vi "GetBooksnAuthors.vi"(0 "reply string":string="150 Opening BINARY mode data connection for directory listing.\r\ntotal 89120\r\n-rw-r--r--  1 rbadmin  staff   11155 Jan 24 23:52 01242009235225_George Chan_Intro to LabVIEW.vi\r\n-rw-r--r--  1 rbadmin  staff  358797 Jan 24 23:52 01242009235225_George Chan_Intro to LabVIEW.zip\r\n-rw-r--r--  1 rbadmin  staff   11154 Jan 25 15:37 01252009153713_Dan Thayer_Intro to LabVIEW.vi\r\n-rw-r--r--  1 rbadmin  staff  368859 Jan 25 15:37 01252009153713_Dan Thayer_Intro to LabVIEW.zip\r\n-rw-r--r--  1 rbadmin  staff   11153 Jan 25 16:41 01252009164134_Dan Thayer_Intro to events.vi\r\n-rw-r--r--  1 rbadmin  staff  373332 Jan 25 16:41 01252009164134_Dan Thayer_Intro to events.zip\r\n-rw-r--r--  1 rbadmin  staff   11200 Jan 25 17:34 01252009173408_Robert Delean_Intro to events.vi\r\n-rw-r--r--  1 rbadmin  staff  337798 Jan 25 17:34 01252009173408_Robert Delean_Intro to events.zip\r\n-rw-r--r--  1 rbadmin  staff   11211 Jan 26 16:19 01262009161919_Alex Brindle_Intro to Events.vi\r\n-rw-r--r--  1 rbadmin  staff  353857 Jan 26 16:19 01262009161919_Alex Brindle_Intro to Events.zip\r\n-rw-r--r--  1 rbadmin  staff   11251 Jan 26 17:08 01262009170754_Alex Brindle_Introduction to LabVIEW.vi\r\n-rw-r--r--  1 rbadmin  staff  356261 Jan 26 17:07 01262009170754_Alex Brindle_Introduction to LabVIEW.zip\r\n-rw-r--r--  1 rbadmin  staff   11251 Jan 26 17:08 01262009170818_Alex Brindle_Introduction to LabVIEW.vi\r\n-rw-r--r--  1 rbadmin  staff  356261 Jan 26 17:08 01262009170818_Alex Brindle_Introduction to LabVIEW.zip\r\n-rw-r--r--  1 rbadmin  staff   11253 Jan 26 17:22 01262009172214_Alex Fernandes_Introduction to LabVIEW.vi\r\n-rw-r--r--  1 rbadmin  staff  355806 Jan 26 17:22 01262009172214_Alex Fernandes_Introduction to LabVIEW.zip\r\n-rw-r--r--  1 rbadmin  staff   11213 Jan 26 17:47 01262009174653_Alex Fernandes_Intro to Events.vi\r\n-rw-r--r--  1 rbadmin  staff  365514 Jan 26 17:46 01262009174653_Alex Fernandes_Intro to Events.zip\r\n-rw-r--r--  1 rbadmin  staff   11237 Jan 26 19:34 01262009193345_Ali Osman_Intro to LabVIEW.vi\r\n-rw-r--r--  1 rbadmin  staff  267924 Jan 26 19:33 01262009193345_Ali Osman_Intro to LabVIEW.zip\r\n-rw-r--r--  1 rbadmin  staff   11219 Jan 26 19:37 01262009193644_Michael Dawson-Haggerty_Intro to LabVIEW.vi\r\n-rw-r--r--  1 rbadmin  staff  268179 Jan 26 19:36 01262009193644_Michael Dawson-Haggerty_Intro to LabVIEW.zip\r\n-rw-r--r--  1 rbadmin  staff   11202 Jan 26 19:59 01262009195911_Michael Dawson-Haggerty_Intro to events.vi\r\n-rw-r--r--  1 rbadmin  staff  314967 Jan 26 19:59 01262009195911_Michael Dawson-Haggerty_Intro to events.zip\r\n-rw-r--r--  1 rbadmin  staff   11236 Jan 26 19:59 01262009195913_Ali Osman_Intro to events.vi\r\n-rw-r--r--  1 rbadmin  staff  315021 Jan 26 19:59 01262009195913_Ali Osman_Intro to events.zip\r\n-rw-r--r--  1 rbadmin  staff   11219 Jan 26 20:18 01262009201827_Timothy Roberts_Intro to LabVIEW.vi\r\n-rw-r--r--  1 rbadmin  staff  317960 Jan 26 20:18 01262009201827_Timothy Roberts_Intro to LabVIEW.zip\r\n-rw-r--r--  1 rbadmin  staff   11250 Jan 26 20:20 01262009202025_Timothy Roberts_Introduction to LabVIEW.vi\r\n-rw-r--r--  1 rbadmin  staff  317960 Jan 26 20:20 01262009202025_Timothy Roberts_Introduction to LabVIEW.zip\r\n-rw-r--r--  1 rbadmin  staff   11250 Jan 26 20:21 01262009202053_Timothy Roberts_Introduction to LabVIEW.vi\r\n-rw-r--r--  1 rbadmin  staff  317960 Jan 26 20:21 01262009202053_Timothy Roberts_Introduction to LabVIEW.zip\r\n-rw-r--r--  1 rbadmin  staff   11184 Jan 26 20:34 01262009203341_Nicole Slaughter_Intro to LabVIEW.vi\r\n-rw-r--r--  1 rbadmin  staff  353125 Jan 26 20:33 01262009203341_Nicole Slaughter_Intro to LabVIEW.zip\r\n-rw-r--r--  1 rbadmin  staff   11224 Jan 26 20:34 01262009203347_Arielle Fakhraee_Intro to LabVIEW.vi\r\n-rw-r--r--  1 rbadmin  staff  362150 Jan 26 20:34 01262009203347_Arielle Fakhraee_Intro to LabVIEW.zip\r\n-rw-r--r--  1 rbadmin  staff   11271 Jan 26 20:35 01262009203457_Arielle Fakhraee_Introduction to LabVIEW.vi\r\n-rw-r--r--  1 rbadmin  staff  362150 Jan 26 20:35 01262009203457_Arielle Fakhraee_Introduction to LabVIEW.zip\r\n-rw-r--r--  1 rbadmin  staff   11227 Jan 26 20:35 01262009203522_Nicole Slaughter_Introduction to LabVIEW.vi\r\n-rw-r--r--  1 rbadmin  staff  353125 Jan 26 20:35 01262009203522_Nicole Slaughter_Introduction to LabVIEW.zip\r\n-rw-r--r--  1 rbadmin  staff   11271 Jan 26 20:36 01262009203528_Arielle Fakhraee_Introduction to LabVIEW.vi\r\n-rw-r--r--  1 rbadmin  staff  362150 Jan 26 20:35 01262009203528_Arielle Fakhraee_Introduction to LabVIEW.zip\r\n-rw-r--r--  1 rbadmin  staff   11231 Jan 26 20:36 01262009203545_Nicole Slaughter_Introduction to LabVIEW.vi\r\n-rw-r--r--  1 rbadmin  staff  353125 Jan 26 20:35 01262009203545_Nicole Slaughter_Introduction to LabVIEW.zip\r\n-rw-r--r--  1 rbadmin  staff   11227 Jan 26 20:36 01262009203608_Nicole Slaughter_Introduction to LabVIEW.vi\r\n-rw-r--r--  1 rbadmin  staff  353125 Jan 26 20:36 01262009203608_Nicole Slaughter_Introduction to LabVIEW.zip\r\n-rw-r--r--  1 rbadmin  staff  321627 Jan 26 20:52 01262009205245_Lawrence Chan_Intro to LabVIEW.zip\r\n-rw-r--r--  1 rbadmin  staff  321661 Jan 26 20:53 01262009205323_Lawrence Chan_Introduction to LabVIEW.zip\r\n-rw-r--r--  1 rbadmin  staff   11248 Jan 26 20:53 01262009205326_Lawrence Chan_Introduction to LabVIEW.vi\r\n-rw-r--r--  1 rbadmin  staff  321661 Jan 26 20:53 01262009205326_Lawrence Chan_Introduction to LabVIEW.zip\r\n-rw-r--r--  1 rbadmin  staff   11201 Jan 26 20:53 01262009205339_Lawrence Chan_Intro to LabVIEW.vi\r\n-rw-r--r--  1 rbadmin  staff  321661 Jan 26 20:53 01262009205339_Lawrence Chan_Intro to LabVIEW.zip\r\n-rw-r--r--  1 rbadmin  staff   11279 Jan 26 21:06 01262009210629_Jeremiah Palmer_Intro to LabVIEW.vi\r\n-rw-r--r--  1 rbadmin  staff  269342 Jan 26 21:06 01262009210629_Jeremiah Palmer_Intro to LabVIEW.zip\r\n-rw-r--r--  1 rbadmin  staff  281166 Jan 26 21:15 01262009211511_William Murphy_Introduction to LabVIEW.zip\r\n-rw-r--r--  1 rbadmin  staff   11202 Jan 26 21:17 01262009211640_William Murphy_Intro to LabVIEW.vi\r\n-rw-r--r--  1 rbadmin  staff  281166 Jan 26 21:17 01262009211640_William Murphy_Intro to LabVIEW.zip\r\n-rw-r--r--  1 rbadmin  staff   11260 Jan 26 21:30 01262009213022_Drew Frankel_Intro to LabVIEW.vi\r\n-rw-r--r--  1 rbadmin  staff  269622 Jan 26 21:30 01262009213022_Drew Frankel_Intro to LabVIEW.zip\r\n-rw-r--r--  1 rbadmin  staff   11202 Jan 26 21:31 01262009213126_Derek Ricciuto_Intro to LabVIEW.vi\r\n-rw-r--r--  1 rbadmin  staff  258314 Jan 26 21:31 01262009213126_Derek Ricciuto_Intro to LabVIEW.zip\r\n-rw-r--r--  1 rbadmin  staff   11155 Jan 26 21:33 01262009213250_Ben Fichera_Intro to LabVIEW.vi\r\n-rw-r--r--  1 rbadmin  staff  264719 Jan 26 21:33 01262009213250_Ben Fichera_Intro to LabVIEW.zip\r\n-rw-r--r--  1 rbadmin  staff   11254 Jan 26 21:45 01262009214517_Timothy Roberts_Introduction to LabVIEW.vi\r\n-rw-r--r--  1 rbadmin  staff  317960 Jan 26 21:45 01262009214517_Timothy Roberts_Introduction to LabVIEW.zip\r\n-rw-r--r--  1 rbadmin  staff   11210 Jan 26 21:46 01262009214556_Timothy Roberts_Intro to Events.vi\r\n-rw-r--r--  1 rbadmin  staff  361042 Jan 26 21:46 01262009214556_Timothy Roberts_Intro to Events.zip\r\n-rw-r--r--  1 rbadmin  staff   11206 Jan 26 21:48 01262009214743_Timothy Roberts_Intro to events.vi\r\n-rw-r--r--  1 rbadmin  staff  361042 Jan 26 21:47 01262009214743_Timothy Roberts_Intro to events.zip\r\n-rw-r--r--  1 rbadmin  staff   11263 Jan 26 22:13 01262009221347_Drew Frankel_Intro to events.vi\r\n-rw-r--r--  1 rbadmin  staff  312829 Jan 26 22:13 01262009221347_Drew Frankel_Intro to events.zip\r\n-rw-r--r--  1 rbadmin  staff   11205 Jan 26 22:14 01262009221419_Derek Ricciuto_Intro to events.vi\r\n-rw-r--r--  1 rbadmin  staff  312573 Jan 26 22:14 01262009221419_Derek Ricciuto_Intro to events.zip\r\n-rw-r--r--  1 rbadmin  staff   11138 Jan 26 22:27 01262009222615_Ben Fichera_Intro to events.vi\r\n-rw-r--r--  1 rbadmin  staff  314194 Jan 26 22:26 01262009222615_Ben Fichera_Intro to events.zip\r\n-rw-r--r--  1 rbadmin  staff   11205 Jan 26 22:44 01262009224413_William Murphy_Intro to events.vi\r\n-rw-r--r--  1 rbadmin  staff  351616 Jan 26 22:44 01262009224413_William Murphy_Intro to events.zip\r\n-rw-r--r--  1 rbadmin  staff   11202 Jan 26 23:01 01262009230112_Courtney Mario_Intro to LabVIEW.vi\r\n-rw-r--r--  1 rbadmin  staff  353710 Jan 26 23:01 01262009230112_Courtney Mario_Intro to LabVIEW.zip\r\n-rw-r--r--  1 rbadmin  staff   11303 Jan 26 23:40 01262009234020_Austin Hsiao_Introduction to LabVIEW.vi\r\n-rw-r--r--  1 rbadmin  staff  283436 Jan 26 23:40 01262009234020_Austin Hsiao_Introduction to LabVIEW.zip\r\n-rw-r--r--  1 rbadmin  staff   11303 Jan 26 23:41 01262009234046_Austin Hsiao_Introduction to LabVIEW.vi\r\n-rw-r--r--  1 rbadmin  staff  283436 Jan 26 23:40 01262009234046_Austin Hsiao_Introduction to LabVIEW.zip\r\n-rw-r--r--  1 rbadmin  staff   11263 Jan 26 23:59 01262009235852_Austin Hsiao_Intro to Events.vi\r\n-rw-r--r--  1 rbadmin  staff  321775 Jan 26 23:59 01262009235852_Austin Hsiao_Intro to Events.zip\r\n-rw-r--r--  1 rbadmin  staff   11266 Jan 27 00:18 01272009001756_Jeremiah Palmer_Intro to events.vi\r\n-rw-r--r--  1 rbadmin  staff  320589 Jan 27 00:18 01272009001756_Jeremiah Palmer_Intro to events.zip\r\n-rw-r--r--  1 rbadmin  staff   11185 Jan 27 01:26 01272009012614_Timothy Li_Intro to Events.vi\r\n-rw-r--r--  1 rbadmin  staff  318752 Jan 27 01:26 01272009012614_Timothy Li_Intro to Events.zip\r\n-rw-r--r--  1 rbadmin  staff   11189 Jan 27 01:42 01272009014223_Taeil Kwak_Intro to events.vi\r\n-rw-r--r--  1 rbadmin  staff  345487 Jan 27 01:42 01272009014223_Taeil Kwak_Intro to events.zip\r\n-rw-r--r--  1 rbadmin  staff   11229 Jan 27 01:52 01272009015247_Timothy Li_Introduction to LabVIEW.vi\r\n-rw-r--r--  1 rbadmin  staff  305926 Jan 27 01:52 01272009015247_Timothy Li_Introduction to LabVIEW.zip\r\n-rw-r--r--  1 rbadmin  staff   11229 Jan 27 01:52 01272009015250_Timothy Li_Introduction to LabVIEW.vi\r\n-rw-r--r--  1 rbadmin  staff  305926 Jan 27 01:52 01272009015250_Timothy Li_Introduction to LabVIEW.zip\r\n-rw-r--r--  1 rbadmin  staff  269378 Jan 27 02:00 01272009020000_Taeil Kwak_Intro to LabVIEW.zip\r\n-rw-r--r--  1 rbadmin  staff   11202 Jan 27 02:10 01272009021016_Courtney Mario_Intro to LabVIEW.vi\r\n-rw-r--r--  1 rbadmin  staff  361928 Jan 27 02:10 01272009021016_Courtney Mario_Intro to LabVIEW.zip\r\n-rw-r--r--  1 rbadmin  staff   11260 Jan 27 04:26 01272009042554_Hannes Daepp_Intro to LabVIEW.vi\r\n-rw-r--r--  1 rbadmin  staff  291101 Jan 27 04:26 01272009042554_Hannes Daepp_Intro to LabVIEW.zip\r\n-rw-r--r--  1 rbadmin  staff   11263 Jan 27 04:32 01272009043213_Hannes Daepp_Intro to events.vi\r\n-rw-r--r--  1 rbadmin  staff  320888 Jan 27 04:32 01272009043213_Hannes Daepp_Intro to events.zip\r\n-rw-r--r--  1 rbadmin  staff   11157 Jan 27 10:09 01272009070920_Andres Cabrera_Intro to Events.vi\r\n-rw-r--r--  1 rbadmin  staff  363534 Jan 27 10:09 01272009070920_Andres Cabrera_Intro to Events.zip\r\n-rw-r--r--  1 rbadmin  staff   11161 Jan 27 10:10 01272009070956_Andres Cabrera_Intro to Events.vi\r\n-rw-r--r--  1 rbadmin  staff  363534 Jan 27 10:10 01272009070956_Andres Cabrera_Intro to Events.zip\r\n-rw-r--r--  1 rbadmin  staff   11157 Jan 27 08:48 01272009084805_Chris Rogers_Problem 1.vi\r\n-rw-r--r--  1 rbadmin  staff  304750 Jan 27 08:48 01272009084805_Chris Rogers_Problem 1.zip\r\n-rw-r--r--  1 rbadmin  staff   11286 Jan 27 09:46 01272009094540_Christopher Martin_Intro to LabVIEW.vi\r\n-rw-r--r--  1 rbadmin  staff  283893 Jan 27 09:45 01272009094540_Christopher Martin_Intro to LabVIEW.zip\r\n-rw-r--r--  1 rbadmin  staff   11285 Jan 27 09:46 01272009094616_Christopher Martin_Intro to events.vi\r\n-rw-r--r--  1 rbadmin  staff  318735 Jan 27 09:46 01272009094616_Christopher Martin_Intro to events.zip\r\n-rw-r--r--  1 rbadmin  staff   11205 Jan 27 12:49 01272009094837_Andres Cabrera_Introduction to LabVIEW.vi\r\n-rw-r--r--  1 rbadmin  staff  288050 Jan 27 12:48 01272009094837_Andres Cabrera_Introduction to LabVIEW.zip\r\n-rw-r--r--  1 rbadmin  staff   11205 Jan 27 12:49 01272009094916_Andres Cabrera_Introduction to LabVIEW.vi\r\n-rw-r--r--  1 rbadmin  staff  288050 Jan 27 12:49 01272009094916_Andres Cabrera_Introduction to LabVIEW.zip\r\n-rw-r--r--  1 rbadmin  staff   11247 Jan 27 13:29 01272009132901_Steve McHugh_Introduction to LabVIEW.vi\r\n-rw-r--r--  1 rbadmin  staff  304519 Jan 27 13:29 01272009132901_Steve McHugh_Introduction to LabVIEW.zip\r\n-rw-r--r--  1 rbadmin  staff   11247 Jan 27 13:29 01272009132924_Steve McHugh_Introduction to LabVIEW.vi\r\n-rw-r--r--  1 rbadmin  staff  304519 Jan 27 13:29 01272009132924_Steve McHugh_Introduction to LabVIEW.zip\r\n-rw-r--r--  1 rbadmin  staff   11247 Jan 27 13:30 01272009132947_Steve McHugh_Introduction to LabVIEW.vi\r\n-rw-r--r--  1 rbadmin  staff  304519 Jan 27 13:29 01272009132947_Steve McHugh_Introduction to LabVIEW.zip\r\n-rw-r--r--  1 rbadmin  staff   11181 Jan 27 14:34 01272009143348_Rachel Yu_Intro to LabVIEW.vi\r\n-rw-r--r--  1 rbadmin  staff  352379 Jan 27 14:34 01272009143348_Rachel Yu_Intro to LabVIEW.zip\r\n-rw-r--r--  1 rbadmin  staff   11180 Jan 27 14:35 01272009143512_Rachel Yu_Intro to events.vi\r\n-rw-r--r--  1 rbadmin  staff  360969 Jan 27 14:35 01272009143512_Rachel Yu_Intro to events.zip\r\n-rw-r--r--  1 rbadmin  staff   11203 Jan 27 14:39 01272009143930_Steve McHugh_Intro to events.vi\r\n-rw-r--r--  1 rbadmin  staff  378401 Jan 27 14:39 01272009143930_Steve McHugh_Intro to events.zip\r\n-rw-r--r--  1 rbadmin  staff   11201 Jan 27 15:49 01272009154908_Robert Delean_Intro to LabVIEW.vi\r\n-rw-r--r--  1 rbadmin  staff  321661 Jan 27 15:49 01272009154908_Robert Delean_Intro to LabVIEW.zip\r\n-rw-r--r--  1 rbadmin  staff   11204 Jan 27 16:15 01272009161523_Lawrence Chan_Intro to events.vi\r\n-rw-r--r--  1 rbadmin  staff  339180 Jan 27 16:15 01272009161523_Lawrence Chan_Intro to events.zip\r\n-rw-r--r--  1 rbadmin  staff   11187 Jan 27 16:32 01272009163211_Nicole Slaughter_Intro to Events.vi\r\n-rw-r--r--  1 rbadmin  staff  397876 Jan 27 16:32 01272009163211_Nicole Slaughter_Intro to Events.zip\r\n-rw-r--r--  1 rbadmin  staff   11183 Jan 27 16:33 01272009163240_Nicole Slaughter_Intro to events.vi\r\n-rw-r--r--  1 rbadmin  staff  397876 Jan 27 16:32 01272009163240_Nicole Slaughter_Intro to events.zip\r\n-rw-r--r--  1 rbadmin  staff   11201 Jan 27 17:41 01272009174122_Allyssa Alair_Intro to LabVIEW.vi\r\n-rw-r--r--  1 rbadmin  staff  268165 Jan 27 17:41 01272009174122_Allyssa Alair_Intro to LabVIEW.zip\r\n-rw-r--r--  1 rbadmin  staff   11223 Jan 27 18:31 01272009183051_Arielle Fakhraee_Intro to events.vi\r\n-rw-r--r--  1 rbadmin  staff  344835 Jan 27 18:31 01272009183051_Arielle Fakhraee_Intro to events.zip\r\n-rw-r--r--  1 rbadmin  staff   11204 Jan 27 19:06 01272009190603_Allyssa Alair_Intro to events.vi\r\n-rw-r--r--  1 rbadmin  staff  341333 Jan 27 19:06 01272009190603_Allyssa Alair_Intro to events.zip\r\n-rw-r--r--  1 rbadmin  staff   11256 Jan 27 19:41 01272009194048_Lindsay Wray_Intro to LabVIEW.vi\r\n-rw-r--r--  1 rbadmin  staff  299707 Jan 27 19:41 01272009194048_Lindsay Wray_Intro to LabVIEW.zip\r\n-rw-r--r--  1 rbadmin  staff   11260 Jan 27 19:44 01272009194344_Lindsay Wray_Intro to events1.vi\r\n-rw-r--r--  1 rbadmin  staff  320787 Jan 27 19:43 01272009194344_Lindsay Wray_Intro to events1.zip\r\n-rw-r--r--  1 rbadmin  staff   11160 Jan 27 20:52 01272009205145_Martin Rosas_Intro to LabVIEW.vi\r\n-rw-r--r--  1 rbadmin  staff  282345 Jan 27 20:51 01272009205145_Martin Rosas_Intro to LabVIEW.zip\r\n-rw-r--r--  1 rbadmin  staff   11184 Jan 27 21:13 01272009211333_Michael Stefaniak_Intro to events.vi\r\n-rw-r--r--  1 rbadmin  staff  317892 Jan 27 21:13 01272009211333_Michael Stefaniak_Intro to events.zip\r\n-rw-r--r--  1 rbadmin  staff  302248 Jan 28 13:20 01282009131958_Winston Lee_Intro to Events.zip\r\n-rw-r--r--  1 rbadmin  staff   11230 Jan 28 13:20 01282009132011_Winston Lee_Introduction to LabVIEW.vi\r\n-rw-r--r--  1 rbadmin  staff  263259 Jan 28 13:20 01282009132011_Winston Lee_Introduction to LabVIEW.zip\r\n-rw-r--r--  1 rbadmin  staff   11254 Jan 29 01:01 01292009010116_Jeremy Fryer-Biggs_Intro to LabVIEW.vi\r\n-rw-r--r--  1 rbadmin  staff  307078 Jan 29 01:01 01292009010116_Jeremy Fryer-Biggs_Intro to LabVIEW.zip\r\n-rw-r--r--  1 rbadmin  staff   11253 Jan 29 01:02 01292009010157_Jeremy Fryer-Biggs_Intro to events.vi\r\n-rw-r--r--  1 rbadmin  staff  373999 Jan 29 01:02 01292009010157_Jeremy Fryer-Biggs_Intro to events.zip\r\n-rw-r--r--  1 rbadmin  staff   11127 Jan 29 11:42 01292009084157_Andres Cabrera_Problem 1.vi\r\n-rw-r--r--  1 rbadmin  staff  319495 Jan 29 11:42 01292009084157_Andres Cabrera_Problem 1.zip\r\n-rw-r--r--  1 rbadmin  staff   11171 Jan 29 11:23 01292009112342_Derek Ricciuto_Problem 1.vi\r\n-rw-r--r--  1 rbadmin  staff  329882 Jan 29 11:23 01292009112342_Derek Ricciuto_Problem 1.zip\r\n-rw-r--r--  1 rbadmin  staff   11171 Jan 29 11:24 01292009112354_Courtney Mario_Problem 1.vi\r\n-rw-r--r--  1 rbadmin  staff  329829 Jan 29 11:24 01292009112354_Courtney Mario_Problem 1.zip\r\n-rw-r--r--  1 rbadmin  staff   11138 Jan 29 11:26 01292009112555_Michael Stefaniak_Problem 1.vi\r\n-rw-r--r--  1 rbadmin  staff  313818 Jan 29 11:26 01292009112555_Michael Stefaniak_Problem 1.zip\r\n-rw-r--r--  1 rbadmin  staff   11234 Jan 29 11:32 01292009113249_Thomas Williamson_Problem 1.vi\r\n-rw-r--r--  1 rbadmin  staff  310150 Jan 29 11:32 01292009113249_Thomas Williamson_Problem 1.zip\r\n-rw-r--r--  1 rbadmin  staff  317133 Jan 29 11:39 01292009113932_Lenny Paritsky_Problem 1.zip\r\n-rw-r--r--  1 rbadmin  staff  317133 Jan 29 11:39 01292009113944_Lenny Paritsky_Problem 1.zip\r\n-rw-r--r--  1 rbadmin  staff  317133 Jan 29 11:40 01292009113956_Lenny Paritsky_Problem 1.zip\r\n-rw-r--r--  1 rbadmin  staff  317133 Jan 29 11:40 01292009114017_Lenny Paritsky_Problem 1.zip\r\n-rw-r--r--  1 rbadmin  staff   11176 Jan 29 11:40 01292009114032_Timothy Roberts_Problem 1.vi\r\n-rw-r--r--  1 rbadmin  staff  333981 Jan 29 11:40 01292009114032_Timothy Roberts_Problem 1.zip\r\n-rw-r--r--  1 rbadmin  staff   11205 Jan 29 11:44 01292009114351_Austin Hsiao_Problem 1.vi\r\n-rw-r--r--  1 rbadmin  staff  319302 Jan 29 11:44 01292009114351_Austin Hsiao_Problem 1.zip\r\n-rw-r--r--  1 rbadmin  staff   11150 Jan 29 12:47 01292009124718_Allyssa Alair_Problem 1.vi\r\n-rw-r--r--  1 rbadmin  staff  313950 Jan 29 12:47 01292009124718_Allyssa Alair_Problem 1.zip\r\n-rw-r--r--  1 rbadmin  staff   11161 Jan 29 13:56 01292009135609_Alex Brindle_Problem 1.vi\r\n-rw-r--r--  1 rbadmin  staff  318222 Jan 29 13:56 01292009135609_Alex Brindle_Problem 1.zip\r\n-rw-r--r--  1 rbadmin  staff   11145 Jan 29 11:27 01292009162717_Steve McHugh_Problem 1.vi\r\n-rw-r--r--  1 rbadmin  staff  324041 Jan 29 11:27 01292009162717_Steve McHugh_Problem 1.zip\r\n-rw-r--r--  1 rbadmin  staff   11145 Jan 29 11:46 01292009164542_Steve McHugh_Problem 1.vi\r\n-rw-r--r--  1 rbadmin  staff  324282 Jan 29 11:46 01292009164542_Steve McHugh_Problem 1.zip\r\n-rw-r--r--  1 rbadmin  staff   11126 Jan 29 16:52 01292009165205_Rachel Yu_Problem 1.vi\r\n-rw-r--r--  1 rbadmin  staff  324303 Jan 29 16:52 01292009165205_Rachel Yu_Problem 1.zip\r\n-rw-r--r--  1 rbadmin  staff   11108 Jan 29 19:03 01292009190317_George Chan_Problem 1.vi\r\n-rw-r--r--  1 rbadmin  staff  319861 Jan 29 19:03 01292009190317_George Chan_Problem 1.zip\r\n-rw-r--r--  1 rbadmin  staff   11122 Jan 29 19:09 01292009190855_George Chan_Intro to events.vi\r\n-rw-r--r--  1 rbadmin  staff  346148 Jan 29 19:09 01292009190855_George Chan_Intro to events.zip\r\n-rw-r--r--  1 rbadmin  staff   11182 Jan 30 10:32 01302009103208_Ali Osman_Problem 1.vi\r\n-rw-r--r--  1 rbadmin  staff  316377 Jan 30 10:32 01302009103208_Ali Osman_Problem 1.zip\r\n-rw-r--r--  1 rbadmin  staff   11285 Jan 30 12:18 01302009121855_Thomas Williamson_Intro to LabVIEW.vi\r\n-rw-r--r--  1 rbadmin  staff  271383 Jan 30 12:18 01302009121855_Thomas Williamson_Intro to LabVIEW.zip\r\n-rw-r--r--  1 rbadmin  staff   11127 Jan 31 19:00 01312009155934_Andres Cabrera_Problem 1.vi\r\n-rw-r--r--  1 rbadmin  staff  327827 Jan 31 18:59 01312009155934_Andres Cabrera_Problem 1.zip\r\n-rw-r--r--  1 rbadmin  staff   11178 Feb  2 01:37 02022009013732_Jeremiah Palmer_HW2.vi\r\n-rw-r--r--  1 rbadmin  staff   97173 Feb  2 01:37 02022009013732_Jeremiah Palmer_HW2.zip\r\n-rw-r--r--  1 rbadmin  staff   11178 Feb  2 01:38 02022009013801_Jeremiah Palmer_HW2.vi\r\n-rw-r--r--  1 rbadmin  staff   97173 Feb  2 01:38 02022009013801_Jeremiah Palmer_HW2.zip\r\n-rw-r--r--  1 rbadmin  staff  318541 Feb  2 03:30 02022009033025_Taeil Kwak_Problem 1.zip\r\n-rw-r--r--  1 rbadmin  staff   11065 Feb  2 18:20 02022009151934_Andres Cabrera_HW2.vi\r\n-rw-r--r--  1 rbadmin  staff   91385 Feb  2 18:19 02022009151934_Andres Cabrera_HW2.zip\r\n-rw-r--r--  1 rbadmin  staff   11121 Feb  2 18:00 02022009180027_Alex Fernandes_HW2.vi\r\n-rw-r--r--  1 rbadmin  staff   90821 Feb  2 18:00 02022009180027_Alex Fernandes_HW2.zip\r\n-rw-r--r--  1 rbadmin  staff   11152 Feb  2 18:16 02022009181607_Ali Osman_HW2.vi\r\n-rw-r--r--  1 rbadmin  staff   90647 Feb  2 18:16 02022009181607_Ali Osman_HW2.zip\r\n-rw-r--r--  1 rbadmin  staff   11057 Feb  2 20:06 02022009200618_Dan Thayer_HW2.vi\r\n-rw-r--r--  1 rbadmin  staff  102182 Feb  2 20:06 02022009200618_Dan Thayer_HW2.zip\r\n-rw-r--r--  1 rbadmin  staff   11113 Feb  2 21:01 02022009210114_William Murphy_HW2.vi\r\n-rw-r--r--  1 rbadmin  staff   90061 Feb  2 21:01 02022009210114_William Murphy_HW2.zip\r\n-rw-r--r--  1 rbadmin  staff   11175 Feb  2 21:23 02022009212311_Austin Hsiao_HW2.vi\r\n-rw-r--r--  1 rbadmin  staff   96865 Feb  2 21:23 02022009212311_Austin Hsiao_HW2.zip\r\n-rw-r--r--  1 rbadmin  staff   11175 Feb  2 21:25 02022009212441_Austin Hsiao_HW2.vi\r\n-rw-r--r--  1 rbadmin  staff   92241 Feb  2 21:24 02022009212441_Austin Hsiao_HW2.zip\r\n-rw-r--r--  1 rbadmin  staff   11123 Feb  2 23:19 02022009231942_Alex Brindle_HW2.vi\r\n-rw-r--r--  1 rbadmin  staff   88591 Feb  2 23:19 02022009231942_Alex Brindle_HW2.zip\r\n-rw-r--r--  1 rbadmin  staff   11122 Feb  2 23:27 02022009232717_Timothy Roberts_HW2.vi\r\n-rw-r--r--  1 rbadmin  staff   95301 Feb  2 23:27 02022009232717_Timothy Roberts_HW2.zip\r\n-rw-r--r--  1 rbadmin  staff   11122 Feb  2 23:28 02022009232740_Timothy Roberts_HW2.vi\r\n-rw-r--r--  1 rbadmin  staff   95301 Feb  2 23:27 02022009232740_Timothy Roberts_HW2.zip\r\n-rw-r--r--  1 rbadmin  staff   11107 Feb  3 00:47 02032009004727_Hannes Daepp_HW2.vi\r\n-rw-r--r--  1 rbadmin  staff   92618 Feb  3 00:47 02032009004727_Hannes Daepp_HW2.zip\r\n-rw-r--r--  1 rbadmin  staff   11148 Feb  3 08:50 02032009085028_Ali Osman_HW2.vi\r\n-rw-r--r--  1 rbadmin  staff   87028 Feb  3 08:50 02032009085028_Ali Osman_HW2.zip\r\n-rw-r--r--  1 rbadmin  staff   11148 Feb  3 08:56 02032009085537_Ali Osman_HW2.vi\r\n-rw-r--r--  1 rbadmin  staff   86748 Feb  3 08:55 02032009085537_Ali Osman_HW2.zip\r\n-rw-r--r--  1 rbadmin  staff   11046 Feb  3 11:58 02032009115758_George Chan_HW2.vi\r\n-rw-r--r--  1 rbadmin  staff   82474 Feb  3 11:58 02032009115758_George Chan_HW2.zip\r\n-rw-r--r--  1 rbadmin  staff   11108 Feb  3 12:00 02032009115956_Lawrence Chan_HW2.vi\r\n-rw-r--r--  1 rbadmin  staff  101803 Feb  3 11:59 02032009115956_Lawrence Chan_HW2.zip\r\n-rw-r--r--  1 rbadmin  staff   11113 Feb  3 13:03 02032009130310_Allyssa Alair_HW21.vi\r\n-rw-r--r--  1 rbadmin  staff   81805 Feb  3 13:03 02032009130310_Allyssa Alair_HW21.zip\r\n-rw-r--r--  1 rbadmin  staff  100380 Feb  3 13:16 02032009131641_Lenny Paritsky_HW2.zip\r\n-rw-r--r--  1 rbadmin  staff   11088 Feb  3 15:35 02032009153445_Rachel Yu_HW2.vi\r\n-rw-r--r--  1 rbadmin  staff  117641 Feb  3 15:35 02032009153445_Rachel Yu_HW2.zip\r\n-rw-r--r--  1 rbadmin  staff   11201 Feb  3 15:36 02032009153613_Christopher Martin_HW2.vi\r\n-rw-r--r--  1 rbadmin  staff   90957 Feb  3 15:36 02032009153613_Christopher Martin_HW2.zip\r\n-rw-r--r--  1 rbadmin  staff   11046 Feb  3 15:48 02032009154723_Ben Fichera_HW2.vi\r\n-rw-r--r--  1 rbadmin  staff   82348 Feb  3 15:48 02032009154723_Ben Fichera_HW2.zip\r\n-rw-r--r--  1 rbadmin  staff   11284 Feb  3 16:02 02032009160215_Thomas Williamson_Intro to events.vi\r\n-rw-r--r--  1 rbadmin  staff  318921 Feb  3 16:02 02032009160215_Thomas Williamson_Intro to events.zip\r\n-rw-r--r--  1 rbadmin  staff   11169 Feb  3 16:11 02032009161108_Jeremy Fryer-Biggs_HW2.vi\r\n-rw-r--r--  1 rbadmin  staff   93692 Feb  3 16:11 02032009161108_Jeremy Fryer-Biggs_HW2.zip\r\n-rw-r--r--  1 rbadmin  staff   11104 Feb  3 16:11 02032009161111_Robert Delean_HW2.vi\r\n-rw-r--r--  1 rbadmin  staff   87086 Feb  3 16:11 02032009161111_Robert Delean_HW2.zip\r\n-rw-r--r--  1 rbadmin  staff   11171 Feb  3 16:31 02032009163115_Lindsay Wray_HW2.vi\r\n-rw-r--r--  1 rbadmin  staff   90645 Feb  3 16:31 02032009163115_Lindsay Wray_HW2.zip\r\n-rw-r--r--  1 rbadmin  staff   11099 Feb  3 17:33 02032009173327_Nicole Slaughter_HW2.vi\r\n-rw-r--r--  1 rbadmin  staff   98920 Feb  3 17:33 02032009173327_Nicole Slaughter_HW2.zip\r\n-rw-r--r--  1 rbadmin  staff  118669 Feb  3 17:44 02032009174347_Arielle Fakhraee_HW2.zip\r\n-rw-r--r--  1 rbadmin  staff   11139 Feb  3 17:45 02032009174523_Arielle Fakhraee_HW2.vi\r\n-rw-r--r--  1 rbadmin  staff  118669 Feb  3 17:45 02032009174523_Arielle Fakhraee_HW2.zip\r\n-rw-r--r--  1 rbadmin  staff   11117 Feb  3 23:38 02032009233759_Courtney Mario_HW2.vi\r\n-rw-r--r--  1 rbadmin  staff   94811 Feb  3 23:38 02032009233759_Courtney Mario_HW2.zip\r\n-rw-r--r--  1 rbadmin  staff   11202 Feb  4 12:32 02042009123143_Lenny Paritsky_Intro to LabVIEW.vi\r\n-rw-r--r--  1 rbadmin  staff  259659 Feb  4 12:32 02042009123143_Lenny Paritsky_Intro to LabVIEW.zip\r\n-rw-r--r--  1 rbadmin  staff   11202 Feb  4 12:33 02042009123257_Lenny Paritsky_Intro to LabVIEW.vi\r\n-rw-r--r--  1 rbadmin  staff  259659 Feb  4 12:33 02042009123257_Lenny Paritsky_Intro to LabVIEW.zip\r\n-rw-r--r--  1 rbadmin  staff   11121 Feb  4 12:37 02042009123637_Lenny Paritsky_HW2.vi\r\n-rw-r--r--  1 rbadmin  staff  100380 Feb  4 12:36 02042009123637_Lenny Paritsky_HW2.zip\r\n-rw-r--r--  1 rbadmin  staff   11205 Feb  4 12:38 02042009123742_Lenny Paritsky_Intro to events.vi\r\n-rw-r--r--  1 rbadmin  staff  346010 Feb  4 12:37 02042009123742_Lenny Paritsky_Intro to events.zip\r\n-rw-r--r--  1 rbadmin  staff   11171 Feb  4 12:39 02042009123847_Lenny Paritsky_Problem 1.vi\r\n-rw-r--r--  1 rbadmin  staff  317133 Feb  4 12:38 02042009123847_Lenny Paritsky_Problem 1.zip\r\n-rw-r--r--  1 rbadmin  staff   11144 Feb  4 15:38 02042009153807_Thomas Williamson_HW2.vi\r\n-rw-r--r--  1 rbadmin  staff   93359 Feb  4 15:38 02042009153807_Thomas Williamson_HW2.zip\r\n-rw-r--r--  1 rbadmin  staff  442949 Feb  5 11:46 02052009114559_Michael Stefaniak_Problem 2.zip\r\n-rw-r--r--  1 rbadmin  staff  442949 Feb  5 11:48 02052009114754_Michael Stefaniak_Problem 2.zip\r\n-rw-r--r--  1 rbadmin  staff   11138 Feb  5 11:54 02052009115402_Michael Stefaniak_Problem 2.vi\r\n-rw-r--r--  1 rbadmin  staff  442949 Feb  5 11:54 02052009115402_Michael Stefaniak_Problem 2.zip\r\n-rw-r--r--  1 rbadmin  staff   11185 Feb  5 11:56 02052009115601_Michael Stefaniak_Intro to LabVIEW.vi\r\n-rw-r--r--  1 rbadmin  staff  296577 Feb  5 11:56 02052009115601_Michael Stefaniak_Intro to LabVIEW.zip\r\n-rw-r--r--  1 rbadmin  staff   11104 Feb  5 11:57 02052009115647_Michael Stefaniak_HW2.vi\r\n-rw-r--r--  1 rbadmin  staff  102096 Feb  5 11:57 02052009115647_Michael Stefaniak_HW2.zip\r\n-rw-r--r--  1 rbadmin  staff   11167 Feb  5 13:06 02052009130648_Derek Ricciuto_Problem 2.vi\r\n-rw-r--r--  1 rbadmin  staff  438034 Feb  5 13:06 02052009130648_Derek Ricciuto_Problem 2.zip\r\n-rw-r--r--  1 rbadmin  staff   11171 Feb  5 13:07 02052009130742_Derek Ricciuto_Problem 2.vi\r\n-rw-r--r--  1 rbadmin  staff  438034 Feb  5 13:07 02052009130742_Derek Ricciuto_Problem 2.zip\r\n-rw-r--r--  1 rbadmin  staff   11182 Feb  5 14:08 02052009140812_Dan Haack_Problem 1.vi\r\n-rw-r--r--  1 rbadmin  staff  308694 Feb  5 14:08 02052009140812_Dan Haack_Problem 1.zip\r\n-rw-r--r--  1 rbadmin  staff   11117 Feb  5 15:57 02052009155742_Derek Ricciuto_HW2.vi\r\n-rw-r--r--  1 rbadmin  staff   90332 Feb  5 15:57 02052009155742_Derek Ricciuto_HW2.zip\r\n-rw-r--r--  1 rbadmin  staff   11126 Feb  5 17:07 02052009170625_Rachel Yu_Problem 2.vi\r\n-rw-r--r--  1 rbadmin  staff  436288 Feb  5 17:07 02052009170625_Rachel Yu_Problem 2.zip\r\n-rw-r--r--  1 rbadmin  staff   11161 Feb  5 18:16 02052009181603_Alex Brindle_Problem 2.vi\r\n-rw-r--r--  1 rbadmin  staff  422180 Feb  5 18:16 02052009181603_Alex Brindle_Problem 2.zip\r\n-rw-r--r--  1 rbadmin  staff   11162 Feb  6 10:33 02062009103301_Peter_Problem 2.vi\r\n-rw-r--r--  1 rbadmin  staff  416209 Feb  6 10:33 02062009103301_Peter_Problem 2.zip\r\n-rw-r--r--  1 rbadmin  staff   11167 Feb  6 15:06 02062009150625_Courtney Mario_Problem 2.vi\r\n-rw-r--r--  1 rbadmin  staff  462742 Feb  6 15:06 02062009150625_Courtney Mario_Problem 2.zip\r\n-rw-r--r--  1 rbadmin  staff   11115 Feb  6 16:29 02062009162931_Steve McHugh_HW2.vi\r\n-rw-r--r--  1 rbadmin  staff   96163 Feb  6 16:29 02062009162931_Steve McHugh_HW2.zip\r\n-rw-r--r--  1 rbadmin  staff   11153 Feb  6 16:34 02062009163349_Steve McHugh_Problem 2.vi\r\n-rw-r--r--  1 rbadmin  staff  436942 Feb  6 16:34 02062009163349_Steve McHugh_Problem 2.zip\r\n-rw-r--r--  1 rbadmin  staff   11153 Feb  6 16:36 02062009163614_Steve McHugh_Problem 2.vi\r\n-rw-r--r--  1 rbadmin  staff  440498 Feb  6 16:36 02062009163614_Steve McHugh_Problem 2.zip\r\n-rw-r--r--  1 rbadmin  staff   11105 Feb  6 17:49 02062009174928_Taeil Kwak_HW2.vi\r\n-rw-r--r--  1 rbadmin  staff   93886 Feb  6 17:49 02062009174928_Taeil Kwak_HW2.zip\r\n") -> (2 "Server Info":T1)   [LabVIEW 2012]
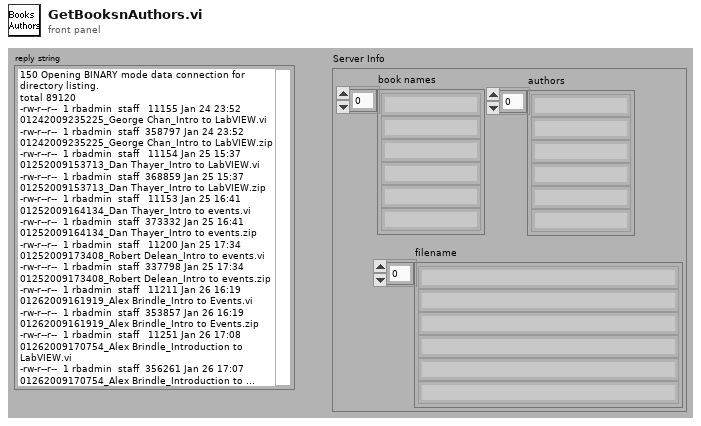
[diagram p1: front panel]
types:
  T1 = cluster{"book names":string[], "authors":string[], "filename":string[]}
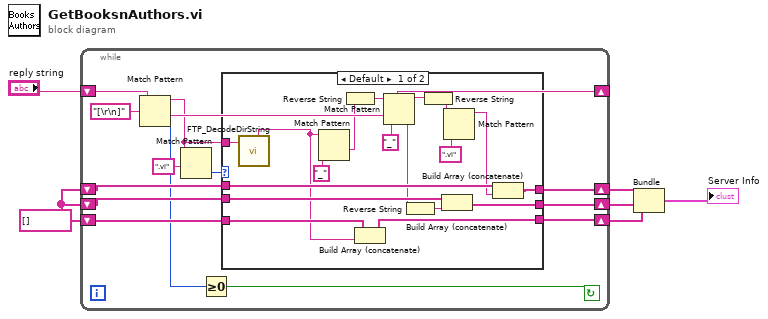
[diagram p0: block diagram]
diagram:
  w5 = string[] []
  n1 = while {
    shift-right: [w18] -> _
    shift-left: "reply string" -> [w20]
    shift-right: [w10] -> w4
    shift-left: w5 -> [w12]
    shift-right: [w9] -> w3
    shift-left: w5 -> [w11]
    shift-right: [w14] -> w2
    shift-left: w5 -> [w15]
    stop <- w7 continue-if-true
    n2 = Match Pattern(string=w20, regular expression="[\r\n]") -> (before substring=w13:string, after substring=w18:string, offset past match=w8:i32)  [unwired: 2 out]
    n3 = Match Pattern(string=w13, regular expression=".vi") -> (offset past match=w16:i32)  [unwired: 4 out]
    n4 = Greater Or Equal To 0?(x=w8) -> (x >= 0?=w7:bool)
    n5 = case shown="Default" w16 {
      tunnel: w15 -> [w38 w41]
      tunnel: [w37 w41] -> w14
      tunnel: w13 -> [w22 _]
      tunnel: w12 -> [w35 w39]
      tunnel: w11 -> [w34 w40]
      tunnel: [w33 w39] -> w10
      tunnel: [w32 w40] -> w9
      frame Default {
        n6 = call <userlib>:"FTP_DecodeDirString.vi"("directory"=w22) -> ("Folder name"=w21:string)  [unwired: 1 in, 5 out]
        n7 = Match Pattern(string=w21, regular expression="_") -> (after substring=w30:string)  [unwired: 4 out]
        n8 = Reverse String(1:w30) -> (0:w27:string)
        n9 = Build Array (concatenate)(w38, w21) -> (w37:string[])
        n10 = Match Pattern(string=w27, regular expression="_") -> (before substring=w24:string, after substring=w25:string)  [unwired: 3 out]
        n11 = Reverse String(1:w25) -> (0:w26:string)
        n12 = Reverse String(1:w24) -> (0:w23:string)
        n13 = Build Array (concatenate)(w34, w26) -> (w32:string[])
        n14 = Match Pattern(string=w23, regular expression=".vi") -> (before substring=w28:string)  [unwired: 4 out]
        n15 = Build Array (concatenate)(w35, w28) -> (w33:string[])
      }
      frame -1 {
      }
    }
  }
  n16 = Bundle(w4, w3, w2) -> (→"Server Info":cluster{string[], string[], string[]})  [unwired: 1 out]
